vi "GEA2 Flash APL.vi"(0 "GEA2 Reference In":refnum<k24>, 2 "Force Update?":bool, 5 "Source Address":u8=228 format="%.0x", 7 "Destination Address":u8 format="%.0x", 9 "File Path":path, 11 "Error In":errorcluster) -> (4 "GEA2 Reference Out":refnum<k24>, 6 "Result":i32(ring) items=["InvalidImage", "ImageRejected", "BoardNotFound", "UnableToGetGeaConfiguration", "WriteToFlashNotAllowed", "ImageDownloadedSuccessfully", "ImagePresent", "WriteToFlashFailed", "EraseFailed", "CrcFailed"], 15 "Error Out":errorcluster)   [LabVIEW 2014, in "GEA2_Toolkit.lvlib"]
doc: "This VI will flash an APL file onto an appliance board. The input 'Filename' accepts a string with file extension, for example 'MC_v1.06.apl'. The APL file must exist in the same directory as the calling VI. Force Update? ensures the APL is downloaded, even if it is the same version as what already exists on the appliance board."
uses:
  library/GEA2_Toolkit.lvlib
  C:/Automation/DLLs/PC Tools .NET/GeaCommunication.dll
  Automation/DLLs/PC Tools .NET/GeaCommunication.dll
  C:/Automation/DLLs/PC Tools .NET/Programming.dll
  Automation/DLLs/PC Tools .NET/Programming.dll
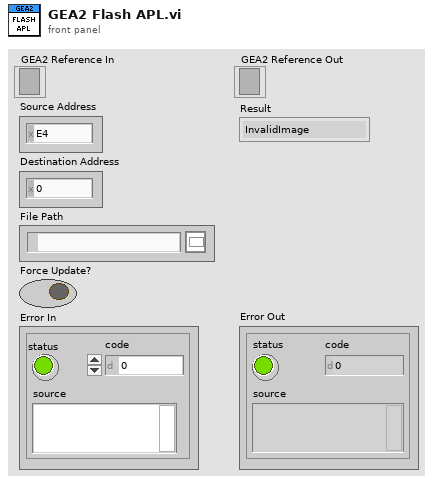
[diagram p1: front panel]
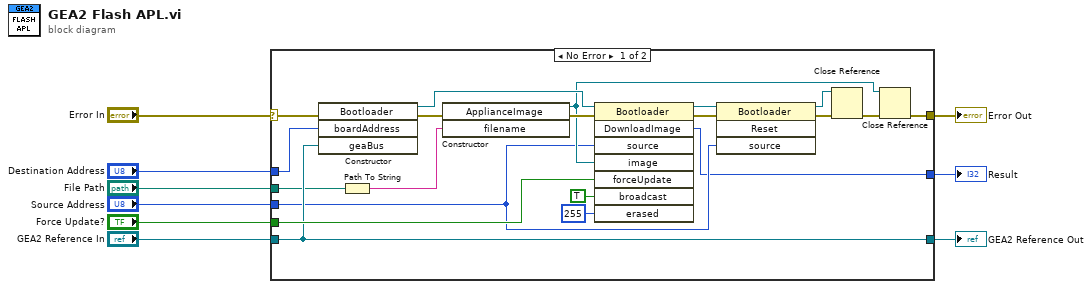
[diagram p0: block diagram]
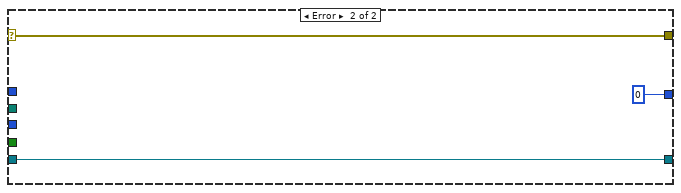
[diagram p2: hidden frame]
diagram:
  n1 = case shown="No Error" "Error In" {
    selector: "Error In" -> [w19 w31]
    tunnel: "GEA2 Reference In" -> [w18 w32]
    tunnel: "Destination Address" -> [w29 _]
    tunnel: "Force Update?" -> [w27 _]
    tunnel: "Source Address" -> [w13 _]
    tunnel: [w12 0 ("DownloadImage")] -> w5
    tunnel: [w20 w31] -> w4
    tunnel: [w18 w32] -> w2
    tunnel: "File Path" -> [w10 _]
    frame No Error {
      n2 = constructor class="Bootloader"(error in=w19, "boardAddress"=w29, "geaBus"=w18) -> (reference out=w24:refnum<k24>, error out=w28:errorcluster)  [unwired: 2 in, 3 out]
      n3 = Path To String(path=w10) -> (string=w11:string)
      n4 = constructor class="ApplianceImage"(error in=w28, "filename"=w11) -> (reference out=w22:refnum<k24>, error out=w25:errorcluster)  [unwired: 2 in, 2 out]
      n5 = invoke class="Bootloader" method="DownloadImage"(reference=w24, error in=w25, "source"=w13, "image"=w22, "forceUpdate"=w27, "broadcast"=TRUE, "erased"=u8 255) -> (reference out=w17:refnum<k24>, error out=w16:errorcluster, "DownloadImage"=w12:i32)  [unwired: 1 in, 5 out]
      n6 = invoke class="Bootloader" method="Reset"(reference=w17, error in=w16, "source"=w13) -> (reference out=w15:refnum<k24>, error out=w14:errorcluster)  [unwired: 1 in, 2 out]
      n7 = Close Reference(reference=w15, error in (no error)=w14) -> (error out=w23:errorcluster)
      n8 = Close Reference(reference=w22, error in (no error)=w23) -> (error out=w20:errorcluster)
    }
    frame Error {
    }
  }
  "GEA2 Reference Out" <- w2
  "Result" <- w5
  "Error Out" <- w4
